vi "VNARP-Read.vi"(0 "ID de connexion":refnum<k5>, 5 "entrée d'erreur (pas d'erreur)":errorcluster, 9 "SIZE":i32=4800) -> (10 "MAGNITUDE 1":sgl[](array[numeric]), 11 "MAGNITUDE 2":sgl[](array[numeric]), 12 "ID de connexion en sortie":refnum<k5>, 13 "sortie d'erreur":errorcluster, 14 "PHASE 1":dbl[](array[numeric]), 16 "ALL DATA":sgl[][](array[numeric]), 17 "DATA":cluster{sgl[], dbl[], sgl[], dbl[]}, 19 "PHASE 2":dbl[](array[numeric]))   [LabVIEW 2021]
uses:
  <vilib>/Analysis/NI_AALPro.lvlib
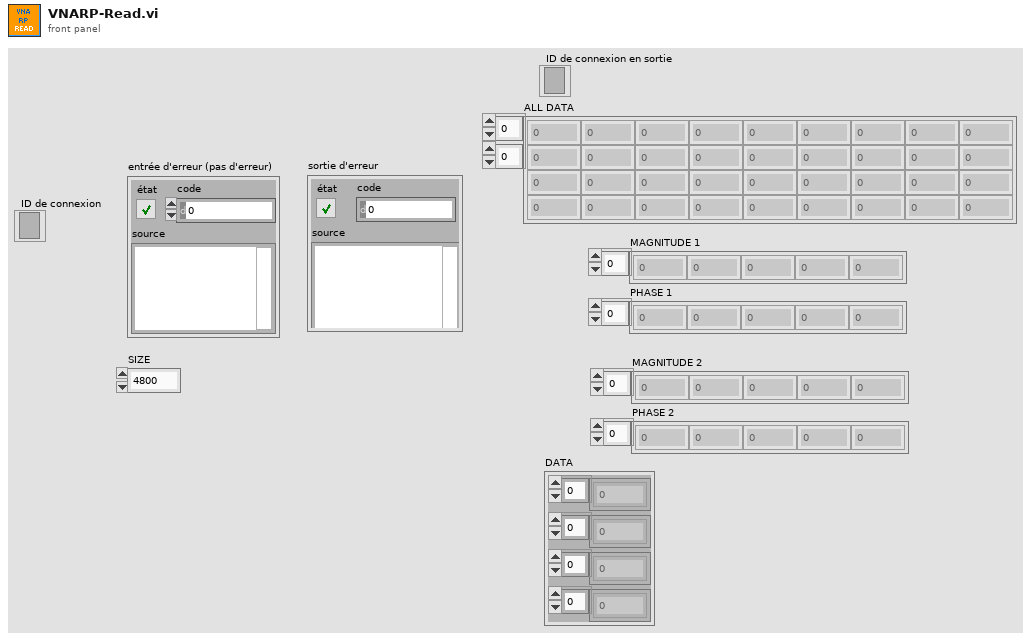
[diagram p1: front panel]
types:
  T1 = enum16{"Standard", "Buffered", "CRLF", "Immediate"}
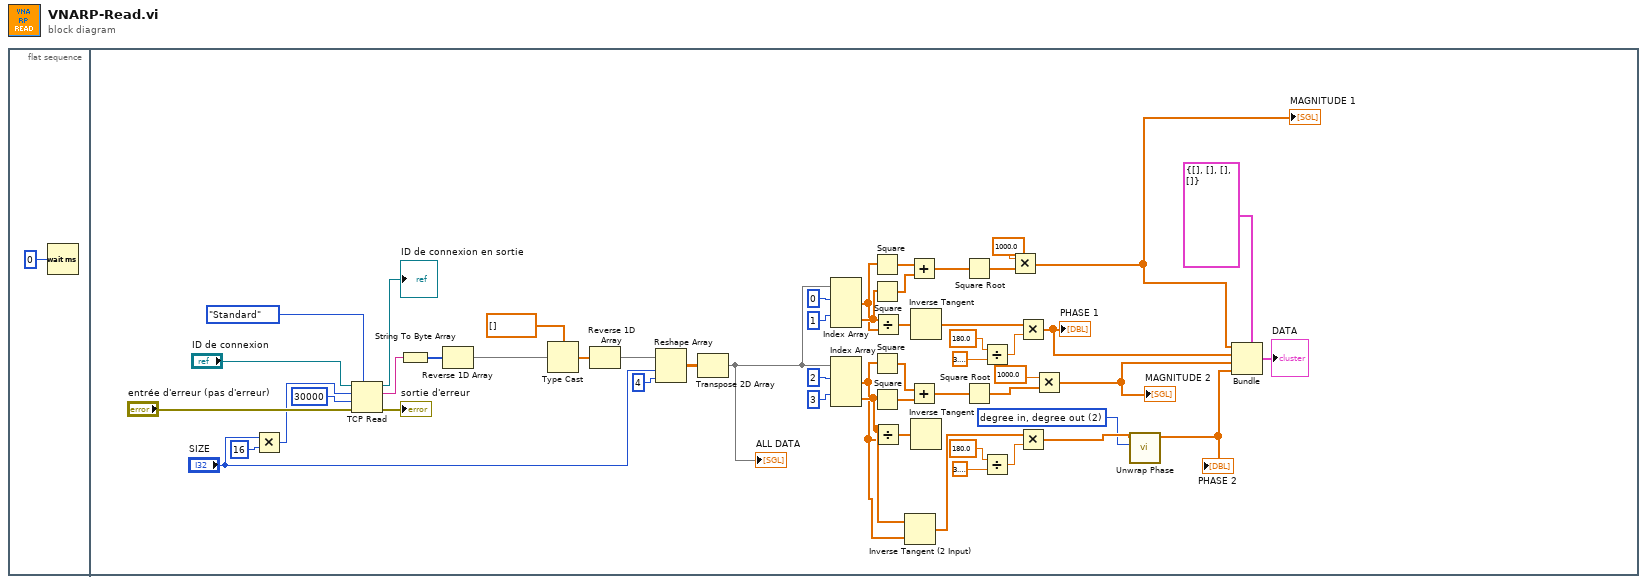
[diagram p0: block diagram]
diagram:
  n1 = flat-sequence {
    frame #0 {
      n2 = Wait (ms)(milliseconds to wait=u32 0 ("attente (ms)")) -> ()  [unwired: 1 out]
    }
    frame #1 {
      w10 = 2 items=["radian in, radian out", "radian in, degree out", "degree in, degree out", "degree in, radian out"] ("phase unit")
      n3 = Multiply(x="SIZE", y=16) -> (x*y=w45:i32)
      n4 = TCP Read(connection ID="ID de connexion", bytes to read=w45, error in (no error)="entrée d'erreur (pas d'erreur)", 7:T1."Standard" ("mode (standard)"), 9:30000 ("timeout en ms (25000)")) -> (connection ID out=→"ID de connexion en sortie":refnum<k5>, data out=w54:string, error out=→"sortie d'erreur":errorcluster)
      n5 = String To Byte Array(string=w54) -> (unsigned byte array=w50:u8[])
      n6 = Reverse 1D Array(array=w50) -> (reversed array=w53:u8[])
      n7 = Type Cast(type=sgl[] [], x=w53) -> (*(type *) &x=w51:sgl[])
      n8 = Reverse 1D Array(array=w51) -> (reversed array=w43:sgl[])
      n9 = Reshape Array(w43, "SIZE", 4 ("taille de la dimension")) -> (w42:sgl[][])
      n10 = Transpose 2D Array(2D array=w42) -> (transposed array=w20:sgl[][])
      "ALL DATA" <- w20
      n11 = Index Array(array=w20, index (row) #1=0 ("indice (ligne)"), index (row) #2=1 ("indice (ligne)")) -> (element #1=w30:sgl[], element #2=w31:sgl[])  [unwired: 2 in]
      n12 = Index Array(array=w20, index (row) #1=2 ("indice (ligne)"), index (row) #2=3 ("indice (ligne)")) -> (element #1=w8:sgl[], element #2=w9:sgl[])  [unwired: 2 in]
      n13 = Square(x=w30) -> (x^2=w39:sgl[])
      n14 = Square(x=w31) -> (x^2=w38:sgl[])
      n15 = Square(x=w8) -> (x^2=w23:sgl[])
      n16 = Square(x=w9) -> (x^2=w24:sgl[])
      n17 = Divide(x=w31, y=w30) -> (x/y=w36:sgl[])
      n18 = Divide(x=w9, y=w8) -> (x/y=w26:sgl[])
      n19 = Inverse Tangent (2 Input)(1:w8, 2:w9) -> (0:w7:sgl[])
      n20 = Add(x=w39, y=w38) -> (x+y=w37:sgl[])
      n21 = Add(x=w23, y=w24) -> (x+y=w25:sgl[])
      n22 = Inverse Tangent(1:w36) -> (0:w35:sgl[])
      n23 = Inverse Tangent(1:w26) -> ()  [unwired: 1 out]
      n24 = Square Root(x=w37) -> (sqrt(x)=w16:sgl[])
      n25 = Square Root(x=w25) -> (sqrt(x)=w2:sgl[])
      n26 = Divide(x=180.0 ("y"), y=3.141592653589793) -> (x/y=w34:dbl)
      n27 = Divide(x=180.0 ("y"), y=3.141592653589793) -> (x/y=w27:dbl)
      n28 = Multiply(x=1000.0 ("y"), y=w16) -> (x*y=w6:dbl[])
      "MAGNITUDE 1" <- w6
      n29 = Multiply(x=w35, y=w34) -> (x*y=w15:dbl[])
      "PHASE 1" <- w15
      n30 = Multiply(x=w7, y=w27) -> (x*y=w12:dbl[])
      n31 = Multiply(x=1000.0 ("y"), y=w2) -> (x*y=w3:dbl[])
      "MAGNITUDE 2" <- w3
      n32 = call <vilib>:"Unwrap Phase.vi"("phase unit"=w10, "Phase"=w12) -> ("Unwrapped Phase"=w11:dbl[])  [unwired: 8 in, 1 out]
      "PHASE 2" <- w11
      n33 = Bundle(cluster=cluster{sgl[], dbl[], sgl[], dbl[]} {[], [], [], []}, w6, w15, w3, w11) -> (→"DATA":cluster{sgl[], dbl[], sgl[], dbl[]})
    }
  }
